vi "Measure.vi"(8 "error in":errorcluster, 11 "FunctionGenerator in":refnum<class "FunctionGenerator.lvclass">) -> (0 "error out":errorcluster, 3 "FunctionGenerator out":refnum<class "FunctionGenerator.lvclass">)   [LabVIEW 2019, in "FunctionGenerator.lvlib" / "FunctionGenerator.lvclass"]
uses:
  Library/FunctionGenerator.lvclass
  Library/FunctionGenerator.lvclass/FunctionGenerator.ctl
  builds/Instruments/Instruments.lvlibp/Library/Instruments.lvclass
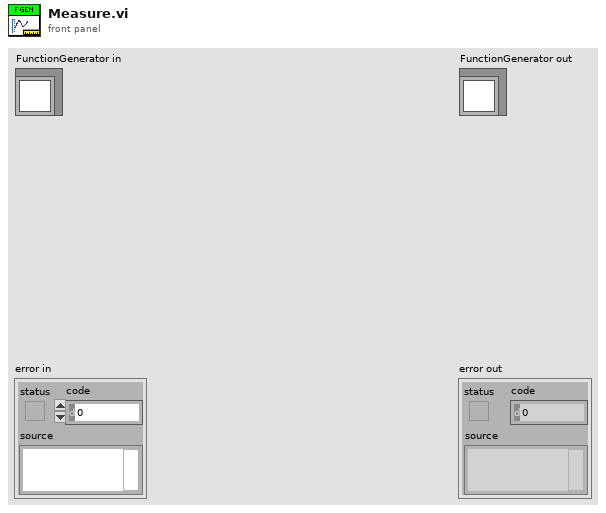
[diagram p1: front panel]
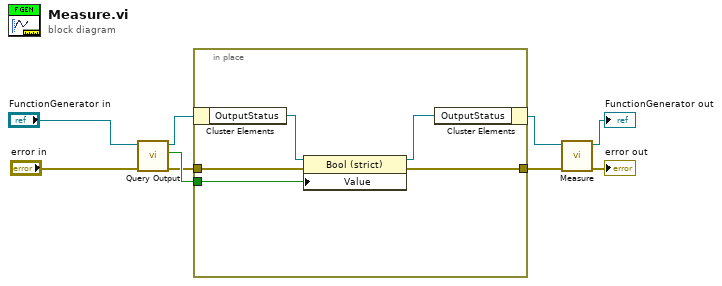
[diagram p0: block diagram]
diagram:
  n1 = call-dynamic "Query Output.vi"("error in (no error)"="error in", "FunctionGenerator in"="FunctionGenerator in") -> ("error out"=w2:errorcluster, "Output"=w4:bool, "FunctionGenerator out"=w5:refnum<class "FunctionGenerator.lvclass">)  [unwired: 7 in]
  n2 = in-place {
    in-place-border: w4 -> [w10]
    in-place-border: w2 -> [w12]
    in-place-border: [w11] -> w1
    n3 = in-place-cluster #1(w5) -> ("OutputStatus"=w14:refnum<vi>)
    n4 = property class="Bool (strict)"(reference=w14, error in=w12, "Value"=w10) -> (reference out=w13:refnum<vi>, error out=w11:errorcluster)
    n5 = in-place-cluster #1("OutputStatus"=w13) -> (w3:refnum<class "FunctionGenerator.lvclass">)
  }
  n6 = call-parent "Measure.vi"("error in"=w1, "Instruments in"=w3) -> ("error out"=→"error out":errorcluster, "Instruments out"=→"FunctionGenerator out":refnum<class "FunctionGenerator.lvclass">)  [unwired: 8 in]
